vi "Continuous Convolution.vi"(7 "algorithm":enum32{"direct", "frequency domain"}(ring)=enum."frequency domain", 8 "init/cont (init:F)":bool, 10 "Kernel":dbl[](array[numeric]), 11 "Array in":dbl[](array[numeric])) -> (0 "error":i32, 3 "Array out":dbl[](array[numeric]))   [LabVIEW 2020, in "NI_MAPro.lvlib"]
uses:
  NI_MAPro.lvlib
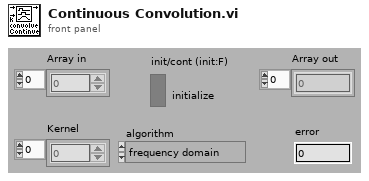
[diagram p1: front panel]
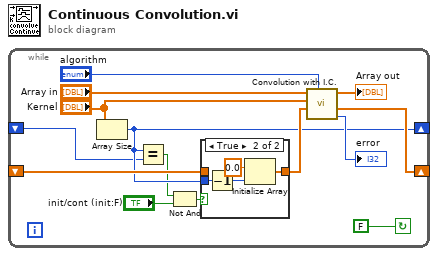
[diagram p0: block diagram]
diagram:
  n1 = while {
    shift-right: [w7] -> _
    shift-left: _ -> [w13]
    shift-right: [w3] -> _
    shift-left: _ -> [w2]
    stop <- FALSE continue-if-true
    n2 = Array Size(array="Kernel") -> (size(s)=w3:i32)
    n3 = Equal?(x=w3, y=w2) -> (x = y?=w1:bool)
    n4 = Not And(1:"init/cont (init:F)", 2:w1) -> (0:w12:bool)
    n5 = case shown="True" w12 {
      tunnel: [w15 w19] -> w9
      tunnel: w13 -> [w15 _]
      tunnel: w3 -> [_ w16]
      frame False {
      }
      frame True {
        n6 = Decrement(x=w16) -> (x-1=w17:i32)
        n7 = Initialize Array(0.0 ("element"), w17) -> (w19:dbl[])
      }
    }
    n8 = call "Convolution with I.C..vi"("algorithm"="algorithm", "Initial conditions"=w9, "Kernel"="Kernel", "Array in"="Array in") -> ("error"=→"error":i32, "final conditions"=w7:dbl[], "Array out"=→"Array out":dbl[])  [unwired: 2 in]
  }
